vi "Verify.vi"(8 "error in (no error)":errorcluster, 9 "Pattern":string, 10 "Mock":refnum<class "Mock.lvclass">, 11 "LUnit Test Case In":refnum<class "Test Case.lvclass">) -> (0 "error out":errorcluster, 3 "LUnit Test Case Out":refnum<class "Test Case.lvclass">)   [LabVIEW 2020, in "String Argument Matching Comparator.lvclass"]
uses:
  String Argument Matching Comparator.lvclass
  Framework/Mock/Mock.lvclass
  <vilib>/Astemes/LUnit/Test Case.lvclass
  C:/git/astemes-lmock/source/Core/Comparator/Comparator.lvclass
  Framework/Verifier/Verifier.lvclass
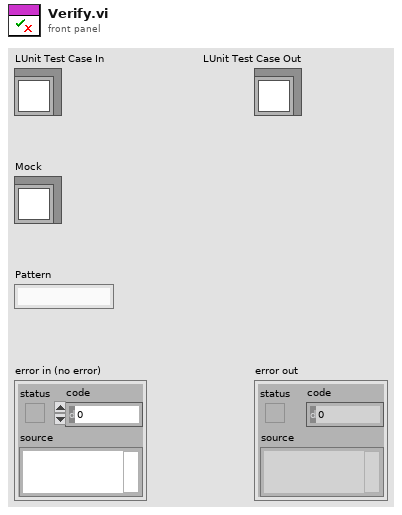
[diagram p1: front panel]
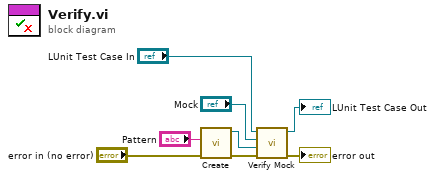
[diagram p0: block diagram]
diagram:
  n1 = call "Create.vi"("error in (no error)"="error in (no error)", "Pattern"="Pattern") -> ("error out"=w6:errorcluster, "String Argument Matching Comparator"=w1:refnum<class "String Argument Matching Comparator.lvclass">)  [unwired: 8 in]
  n2 = call "Verify Mock.vi"("error in (no error)"=w6, "Comparator"=w1, "Mock"="Mock", "LUnit Test Case In"="LUnit Test Case In") -> ("error out"=→"error out":errorcluster, "LUnit Test Case Out"=→"LUnit Test Case Out":refnum<class "Test Case.lvclass">)  [unwired: 6 in]
